vi "LoadTree.vi"(8 "error in":errorcluster, 10 "Horizontal Graduated Bar 2":refnum<vi>, 11 "TreeControl reference":refnum<vi>) -> (0 "error out":errorcluster)   [LabVIEW 2014]
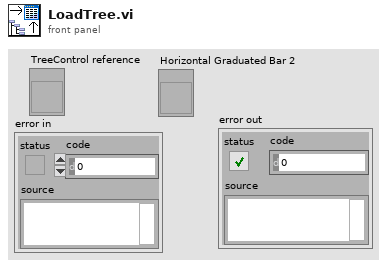
[diagram p1: front panel]
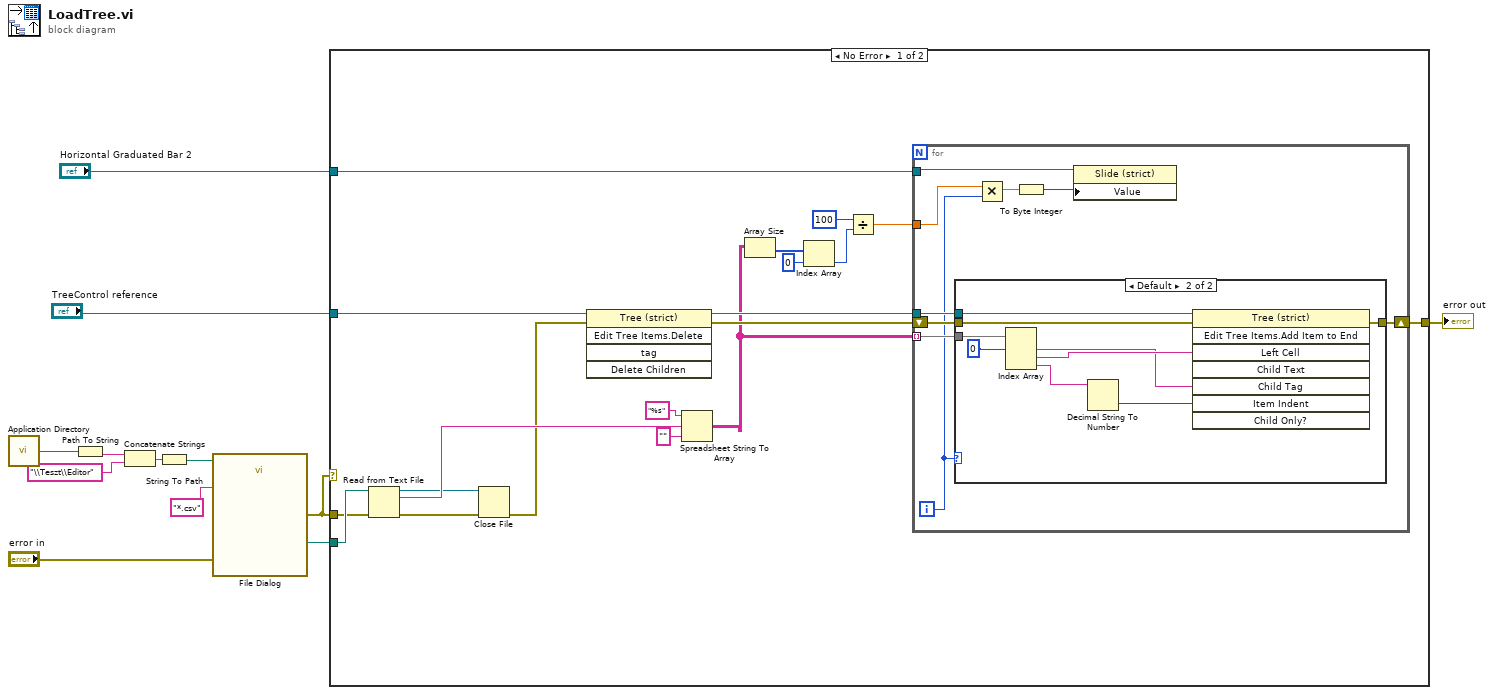
[diagram p0: block diagram]
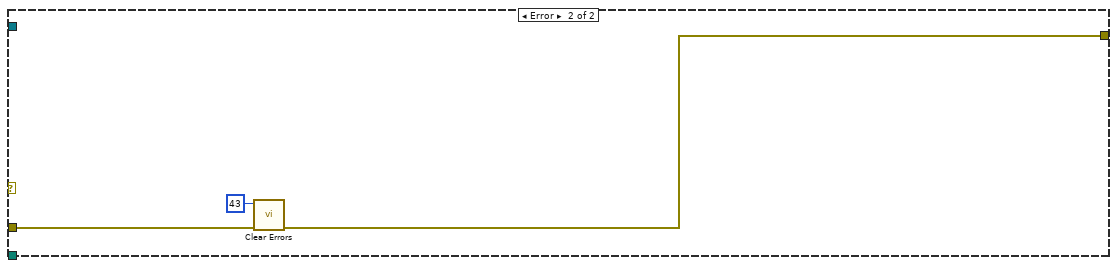
[diagram p3: hidden frame]
diagram:
  n1 = call <vilib>:"Application Directory.vi"() -> ("Application Directory"=w6:path)
  n2 = Path To String(path=w6) -> (string=w10:string)
  n3 = Concatenate Strings(w10, "\\Teszt\\Editor" ("prompt (Choose or enter file path)")) -> (w9:string)
  n4 = String To Path(string=w9) -> (path=w7:path)
  n5 = call "File Dialog"("start path"=w7, "error in"="error in", "pattern (all files)"="*.csv") -> ("selected path"=w5:path, "error out"=w2:errorcluster)  [unwired: 9 in, 2 out]
  n6 = case shown="No Error" w2 {
    tunnel: "TreeControl reference" -> [w30 _]
    tunnel: w5 -> [w22 _]
    tunnel: w2 -> [w21 w53]
    tunnel: [w20 w52] -> w3
    tunnel: "Horizontal Graduated Bar 2" -> [w15 _]
    frame No Error {
      n7 = Read from Text File(file (use dialog)=w22, error in=w21) -> (refnum out=w25:refnum<file>, text=w27:string, error out=w24:errorcluster)  [unwired: 1 in, 2 out]
      n8 = Close File(refnum=w25, error in=w24) -> (error out=w26:errorcluster)  [unwired: 1 out]
      n9 = invoke on="Invoke Node" class="Tree (strict)" method="Edit Tree Items.Delete"(reference=w30, error in=w26) -> (reference out=w31:refnum<vi>, error out=w29:errorcluster)  [unwired: 3 in, 3 out]
      n10 = Spreadsheet String To Array(format string="%s", spreadsheet string=w27, array type (2D Dbl)="") -> (array=w19:string[][])  [unwired: 1 in]
      n11 = Array Size(array=w19) -> (size(s)=w18:i32[])
      n12 = Index Array(array=w18, index=0) -> (element=w16:i32)
      n13 = Divide(x=100, y=w16) -> (x/y=w13:dbl)
      n14 = for {
        tunnel: w31 -> [w40]
        tunnel: w19 -> [w38] mode=indexing
        shift-right: [w39] -> w20
        shift-left: w29 -> [w36]
        tunnel: w15 -> [w37]
        tunnel: w13 -> [w34]
        i -> [w35]
        n15 = case shown="Default" w35 {
          tunnel: w40 -> [_ w48]
          tunnel: w36 -> [w41 w47]
          tunnel: [w41 w46] -> w39
          tunnel: w38 -> [_ w44]
          frame 0 {
            # "fejlécet eldobjuk"
          }
          frame Default {
            n16 = Index Array(array=w44, index #1=0 ("index")) -> (element #1=w42:string, element #2=w43:string, element #3=w45:string)  [unwired: 2 in]
            n17 = Decimal String To Number(string=w45) -> (number=w49:i32)  [unwired: 2 in, 1 out]
            n18 = invoke on="Invoke Node" class="Tree (strict)" method="Edit Tree Items.Add Item to End"(reference=w48, error in=w47, "Left Cell"=w43, "Child Tag"=w42, "Item Indent"=w49) -> (error out=w46:errorcluster)  [unwired: 3 in, 7 out]
          }
        }
        n19 = Multiply(x=w34, y=w35) -> (x*y=w33:dbl)
        n20 = To Byte Integer(number=w33) -> (8bit integer=w32:i8)
        n21 = property class="Slide (strict)"(reference=w37, "Value"=w32) -> ()  [unwired: 1 in, 2 out]
      }
    }
    frame Error {
      n22 = call <vilib>:"Clear Errors.vi"("error in (no error)"=w53, "specific error code to clear (0: all)"=43) -> ("error out"=w52:errorcluster)  [unwired: 4 in, 1 out]
    }
  }
  "error out" <- w3
